vi "Get File Paths.vi"() -> (2 "Test Profiles Directory":path, 3 "Settings Path":path)   [LabVIEW 2018]
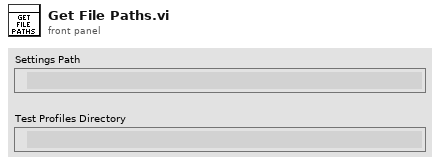
[diagram p1: front panel]
types:
  T1 = enum32{"invalid app kind", "Development System", "Run Time System", "Student Edition", "Embedded LabVIEW", "Evaluation", "Custom"}
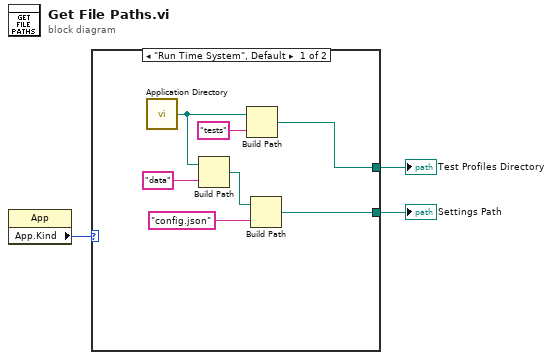
[diagram p0: block diagram]
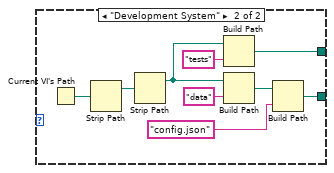
[diagram p2: hidden frame]
diagram:
  n1 = property class="App"() -> ("App.Kind"=w3:T1)  [unwired: 2 in, 2 out]
  n2 = case shown="\"Run Time System\", Default" w3 {
    tunnel: [w7 w14] -> w2
    tunnel: [w4 w11] -> w1
    frame "Run Time System", Default {
      n3 = call <vilib>:"Application Directory.vi"() -> ("Application Directory"=w6:path)
      n4 = Build Path(base path=w6, name or relative path="data") -> (appended path=w9:path)
      n5 = Build Path(base path=w6, name or relative path="tests") -> (appended path=w4:path)
      n6 = Build Path(base path=w9, name or relative path="config.json") -> (appended path=w7:path)
    }
    frame "Development System" {
      n7 = Current VI's Path() -> (path=w19:path)
      n8 = Strip Path(path=w19) -> (stripped path=w18:path)  [unwired: 1 out]
      n9 = Strip Path(path=w18) -> (stripped path=w12:path)  [unwired: 1 out]
      n10 = Build Path(base path=w12, name or relative path="tests") -> (appended path=w11:path)
      n11 = Build Path(base path=w12, name or relative path="data") -> (appended path=w16:path)
      n12 = Build Path(base path=w16, name or relative path="config.json") -> (appended path=w14:path)
    }
  }
  "Settings Path" <- w2
  "Test Profiles Directory" <- w1
